vi "Read Flow Control Valve Setpoint.vi"(11 "IActuatorCylinder in":refnum<class "ILCControlledActuatorCylinder.lvclass">) -> (2 "Flow Control Valve Setpoint":dbl[unit], 3 "IActuatorCylinder out":refnum<class "ILCControlledActuatorCylinder.lvclass">)   [LabVIEW 2015, in "ILCControlledActuatorCylinder.lvclass"]
uses:
  ILCControlledActuatorCylinder.lvclass
  ILCControlledActuatorCylinder.lvclass/ILCControlledActuatorCylinder.ctl
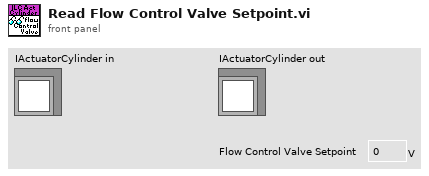
[diagram p1: front panel]
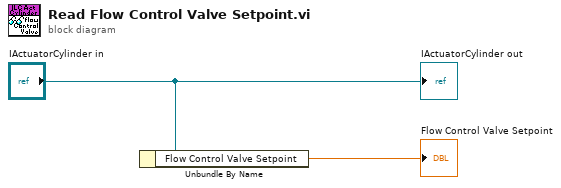
[diagram p0: block diagram]
diagram:
  n1 = Unbundle By Name("IActuatorCylinder in") -> ("Flow Control Valve Setpoint"=→"Flow Control Valve Setpoint":dbl[unit])
  "IActuatorCylinder out" <- "IActuatorCylinder in"
